vi "Set Window Origin.vi"(0 "VI in":refnum<vi>, 7 "Origin":T1, 11 "error in (no error)":errorcluster) -> (4 "VI out":refnum<vi>, 6 "pane":refnum<vi>, 15 "error out":errorcluster)   [LabVIEW 2020]
uses:
  <vilib>/Utility/miscctls.llb/LVPointTypeDef.ctl
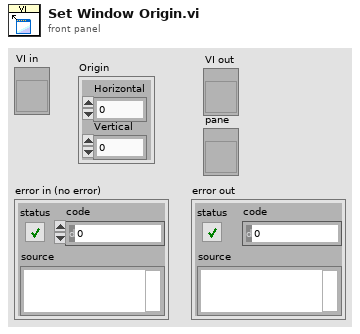
[diagram p1: front panel]
types:
  T1 = typedef "LVPointTypeDef.ctl" = cluster{"Horizontal":i16, "Vertical":i16}
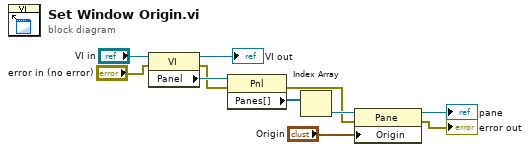
[diagram p0: block diagram]
diagram:
  n1 = property class="VI"(reference="VI in", error in="error in (no error)") -> (reference out=→"VI out":refnum<vi>, error out=w2:errorcluster, "Panel"=w9:refnum<vi>)
  n2 = property class="Pnl"(reference=w9, error in=w2) -> (error out=w6:errorcluster, "Panes[]"=w8:refnum<vi>[])  [unwired: 1 out]
  n3 = Index Array(array=w8) -> (element=w7:refnum<vi>)  [unwired: 1 in]
  n4 = property class="Pane"(reference=w7, error in=w6, "Origin"="Origin") -> (reference out=→"pane":refnum<vi>, error out=→"error out":errorcluster)
